vi "Set Unit to degC.vi"(8 "error in":errorcluster, 11 "TE Cooler in":refnum<class "TE Cooler.lvclass">) -> (0 "error out":errorcluster, 3 "TE Cooler out":refnum<class "TE Cooler.lvclass">)   [LabVIEW 2015, in "TE Cooler.lvlib" / "TE Cooler.lvclass"]
uses:
  TE Cooler.lvclass
  Controls/Command.ctl
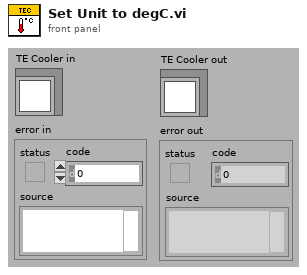
[diagram p1: front panel]
types:
  T1 = typedef "TE Cooler.lvlib/TE Cooler.lvclass/Command.ctl" = enum16{"INPUT1", "DESIRED CONTROL VALUE", "POWER OUTPUT", "ALARM STATUS", "INPUT 2", "OUTPUT CURRENT COUNTS", "ALARM TYPE", "SET TYPE DEFINE", "SENSOR TYPE", "CONTROL TYPE", "CONTROL OUTPUT POLARITY", "POWER ON/OFF", "OUTPUT SHUTDOWN IF ALARM", "FIXED DESIRED CONTROL SETTING", "PROPORTIONAL BANDWIDTH", "INTEGRAL GAIN", "DERIVATIVE GAIN", "LOW EXTERNAL SET RANGE", "HIGH EXTERNAL SET RANGE", "ALARM DEADBAND", "HIGH ALARM SETTING", "LOW ALARM SETTING", "CONTROL DEADBAND SETTING", "INPUT1 OFFSET", "INPUT2 OFFSET", "HEAT MULTIPLIER", "COOL MULTIPLIER", "OVER CURRENT COUNT COMPARE VALUE", "ALARM LATCH ENABLE", "NOT USED", "ALARM LATCH RESET", "CHOOSE SENSOR FOR ALARM FUNCTION", "CHOOSE TEMPERATURE WORKING UNITS", "EEPROM WRITE ENABLE", "OVER CURRENT CONTINUOUS", "OVER CURRENT RESTART ATTEMPTS", "JP3 DISPLAY ENABLE"}
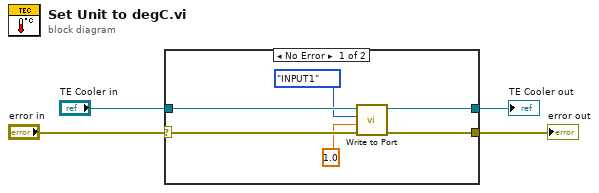
[diagram p0: block diagram]
diagram:
  n1 = case shown="No Error" "error in" {
    selector: "error in" -> [w8 w12]
    tunnel: [w7 w12] -> w3
    tunnel: [w9 w11] -> w1
    tunnel: "TE Cooler in" -> [w10 w11]
    frame No Error {
      n2 = call "Write to Port.vi"("error in"=w8, "Input Value"=1.0, "TEC Cmd"=Command."INPUT1", "TE Cooler in"=w10) -> ("error out"=w7:errorcluster, "TE Cooler out"=w9:refnum<class "TE Cooler.lvclass">)  [unwired: 5 in, 1 out]
    }
    frame Error {
    }
  }
  "error out" <- w3
  "TE Cooler out" <- w1
